vi "ListenPort.vi"(7 "IsEnabled":bool, 8 "error constant":errorcluster, 9 "StopThread":bool, 10 "IsCamera":bool, 11 "Port":u16) -> (0 "error out":errorcluster, 1 "Socket Closed":bool, 2 "OutBytes":u8[](array[numeric]), 3 "OutString":string)   [LabVIEW 2019]
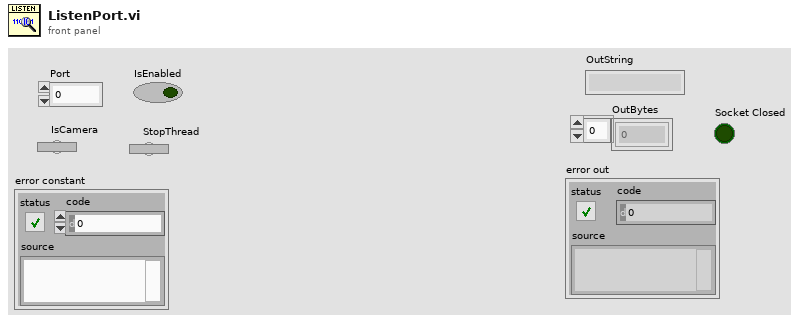
[diagram p1: front panel]
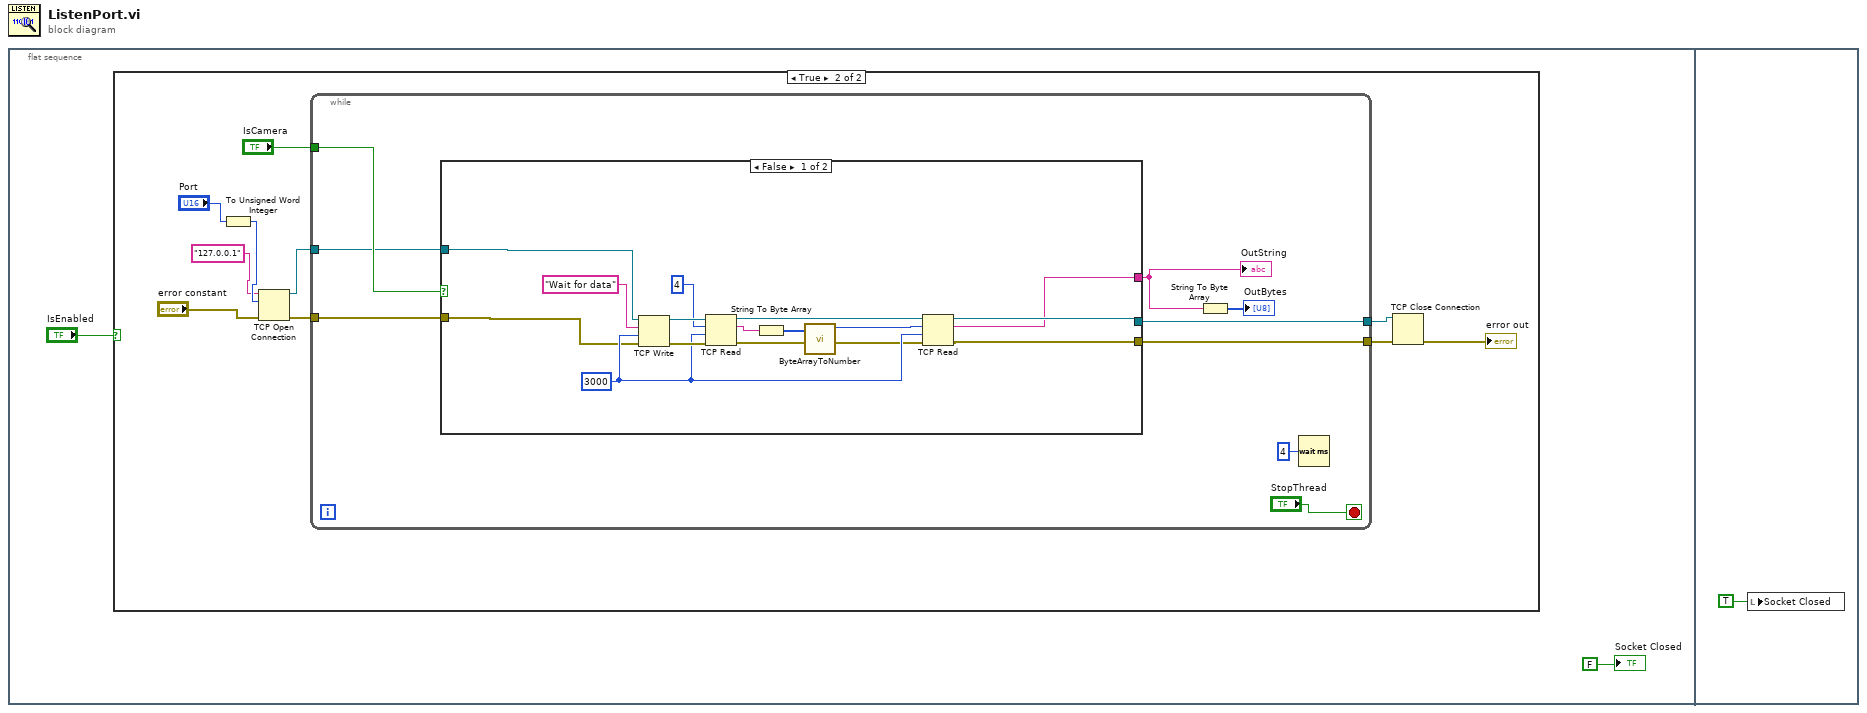
[diagram p0: block diagram]
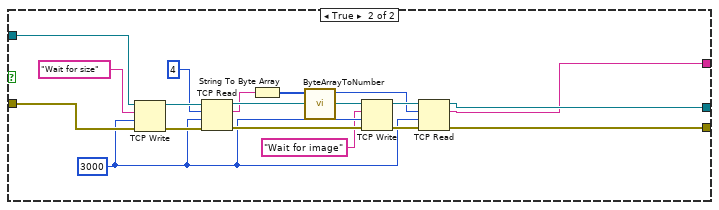
[diagram p3: hidden frame]
diagram:
  n1 = flat-sequence {
    frame #0 {
      n2 = case shown="True" "IsEnabled" {
        frame False {
        }
        frame True {
          n3 = To Unsigned Word Integer(number="Port") -> (unsigned 16bit integer=w5:u16)
          n4 = TCP Open Connection(address="127.0.0.1", remote port or service name=w5, error in (no error)="error constant") -> (connection ID=w10:refnum<k5>, error out=w8:errorcluster)  [unwired: 2 in]
          n5 = while {
            tunnel: "IsCamera" -> [w19]
            tunnel: w8 -> [w18]
            tunnel: [w17] -> w9
            tunnel: w10 -> [w15]
            tunnel: [w14] -> w11
            stop <- "StopThread" stop-if-true
            n6 = case shown="False" w19 {
              tunnel: w18 -> [w30 w53]
              tunnel: [w29 w46] -> w17
              tunnel: w15 -> [w31 w52]
              tunnel: [w25 w47] -> w14
              tunnel: [w24 w39] -> w13
              frame False {
                w33 = 3000 ("timeout ms (25000)")
                n7 = TCP Write(connection ID=w31, data in="Wait for data", error in (no error)=w30, 9:w33) -> (connection ID out=w35:refnum<k5>, error out=w36:errorcluster)  [unwired: 1 out]
                n8 = TCP Read(connection ID=w35, bytes to read=4, error in (no error)=w36, 9:w33) -> (connection ID out=w27:refnum<k5>, data out=w26:string, error out=w28:errorcluster)  [unwired: 1 in]
                n9 = String To Byte Array(string=w26) -> (unsigned byte array=w23:u8[])
                n10 = call "ByteArrayToNumber.vi"("In Array"=w23) -> ("Out Number"=w22:u32)  [unwired: 10 in]
                n11 = TCP Read(connection ID=w27, bytes to read=w22, error in (no error)=w28, 9:w33) -> (connection ID out=w25:refnum<k5>, data out=w24:string, error out=w29:errorcluster)  [unwired: 1 in]
              }
              frame True {
                w43 = 3000 ("timeout ms (25000)")
                n12 = TCP Write(connection ID=w52, data in="Wait for size", error in (no error)=w53, 9:w43) -> (connection ID out=w51:refnum<k5>, error out=w54:errorcluster)  [unwired: 1 out]
                n13 = TCP Read(connection ID=w51, bytes to read=4, error in (no error)=w54, 9:w43) -> (connection ID out=w49:refnum<k5>, data out=w41:string, error out=w44:errorcluster)  [unwired: 1 in]
                n14 = String To Byte Array(string=w41) -> (unsigned byte array=w38:u8[])
                n15 = call "ByteArrayToNumber.vi"("In Array"=w38) -> ("Out Number"=w37:u32)  [unwired: 10 in]
                n16 = TCP Write(connection ID=w49, data in="Wait for image", error in (no error)=w44, 9:w43) -> (connection ID out=w48:refnum<k5>, error out=w45:errorcluster)  [unwired: 1 out]
                n17 = TCP Read(connection ID=w48, bytes to read=w37, error in (no error)=w45, 9:w43) -> (connection ID out=w47:refnum<k5>, data out=w39:string, error out=w46:errorcluster)  [unwired: 1 in]
              }
            }
            "OutString" <- w13
            n18 = String To Byte Array(string=w13) -> (unsigned byte array=→"OutBytes":u8[])
            n19 = Wait (ms)(milliseconds to wait=u32 4) -> ()  [unwired: 1 out]
          }
          n20 = TCP Close Connection(connection ID=w11, error in (no error)=w9) -> (error out=→"error out":errorcluster)  [unwired: 1 in, 1 out]
        }
      }
      "Socket Closed" <- FALSE
    }
    frame #1 {
      n21 = local write "Socket Closed"(TRUE) -> ()
    }
  }
